vi "PID_Separate(subvi).vi"(6 "Vasen":dbl format="%.2f", 7 "Oikea":dbl format="%.2f", 9 "Reset Encoders":bool, 10 "Taka":dbl format="%.2f", 11 "Etu":dbl format="%.2f") -> ()   [LabVIEW 2018]
uses:
  <vilib>/addons/control/pid/NI_PID_pid.lvlib
  <vilib>/addons/control/pid/pid.llb/PID (DBL).vi
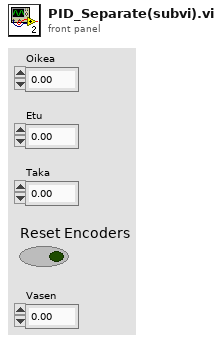
[diagram p1: front panel]
types:
  T1 = cluster{bool, "Tick Count(uSec)":u32, "Counter Value":i32[], "x-y":i32[]}
  T2 = cluster{"Position":i32[], "Velocity RPM":dbl[], "Velocity RPS":dbl[], "Radians/s":dbl[]}
  T3 = cluster{"proportional gain (Kc)":dbl, "integral time (Ti, min)":dbl, "derivative time (Td, min)":dbl}
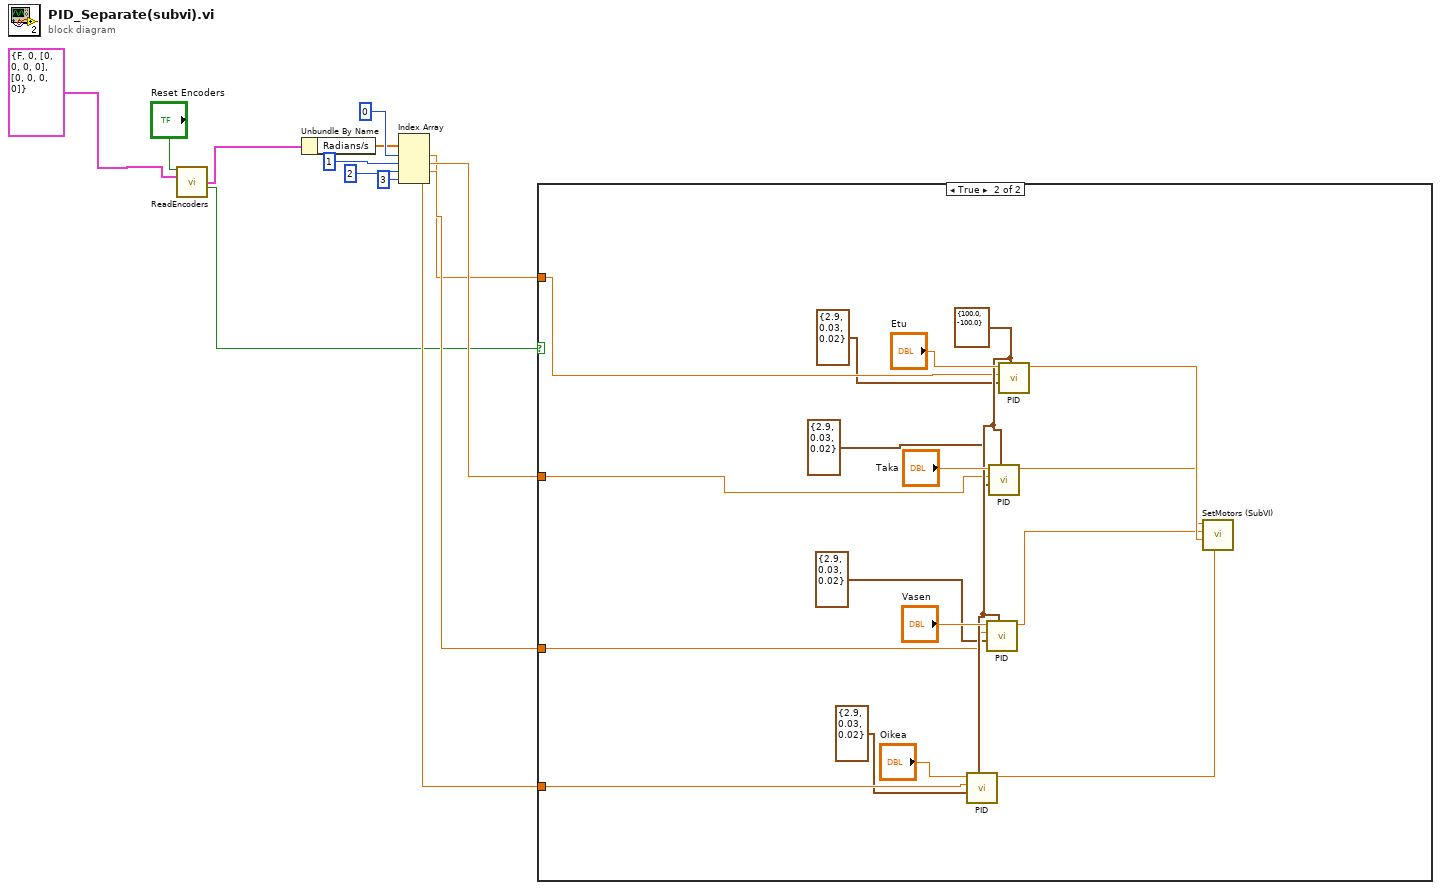
[diagram p0: block diagram]
diagram:
  n1 = call "ReadEncoders.vi"("Reset Encoders"="Reset Encoders", "Cluster in"=T1 {FALSE, "Tick Count(uSec)"=0, "Counter Value"=[0, 0, 0, 0], "x-y"=[0, 0, 0, 0]}) -> ("output cluster"=w4:T2, "Updated"=w2:bool)  [unwired: 9 in, 3 out]
  n2 = Unbundle By Name(w4) -> ("Radians/s"=w5:dbl[])
  n3 = Index Array(array=w5, index #1=0 ("index"), index #2=1 ("index"), index #3=2 ("index"), index #4=3 ("index")) -> (element #1=w6:dbl, element #2=w7:dbl, element #3=w8:dbl, element #4=w9:dbl)
  n4 = case shown="True" w2 {
    tunnel: w6 -> [_ w21]
    tunnel: w7 -> [_ w20]
    tunnel: w8 -> [_ w19]
    tunnel: w9 -> [_ w18]
    frame False {
    }
    frame True {
      w22 = cluster{"output high":dbl, "output low":dbl} {"output high"=100.0, "output low"=-100.0} ("output range")
      n5 = call-poly <vilib>:"PID.vi"("output range"=w22, "PID gains"=T3 {"proportional gain (Kc)"=2.9, "integral time (Ti, min)"=0.03, "derivative time (Td, min)"=0.02}, "process variable"=w18, "setpoint"="Oikea") -> ("output"=w23:dbl)  [unwired: 6 in, 1 out]
      n6 = call-poly <vilib>:"PID.vi"("output range"=w22, "PID gains"=T3 {"proportional gain (Kc)"=2.9, "integral time (Ti, min)"=0.03, "derivative time (Td, min)"=0.02}, "process variable"=w19, "setpoint"="Vasen") -> ("output"=w24:dbl)  [unwired: 6 in, 1 out]
      n7 = call-poly <vilib>:"PID.vi"("output range"=w22, "PID gains"=T3 {"proportional gain (Kc)"=2.9, "integral time (Ti, min)"=0.03, "derivative time (Td, min)"=0.02}, "process variable"=w20, "setpoint"="Taka") -> ("output"=w25:dbl)  [unwired: 6 in, 1 out]
      n8 = call-poly <vilib>:"PID.vi"("output range"=w22, "PID gains"=T3 {"proportional gain (Kc)"=2.9, "integral time (Ti, min)"=0.03, "derivative time (Td, min)"=0.02}, "process variable"=w21, "setpoint"="Etu") -> ("output"=w26:dbl)  [unwired: 6 in, 1 out]
      n9 = call "SetMotors (SubVI).vi"("Oikea"=w23, "Etu"=w26, "Vasen"=w24, "Taka"=w25) -> ()  [unwired: 8 in]
    }
  }
